vi "Encoder Init.vi"(0 "Portas":T1={"Acionador"="Dev1/port0/line7", "Clock"="Dev1/ctr0", "Canal Analogico"="Dev1/ai22", "Trigger"="/Dev1/PFI11"}) -> (3 "Task Out":T2, 6 "error out":errorcluster)   [LabVIEW 2019]
uses:
  <vilib>/DAQmx/create/channels.llb/DAQmx Create Channel (AI-Voltage-Basic).vi
  <vilib>/DAQmx/configure/timing.llb/DAQmx Timing (Sample Clock).vi
  <vilib>/DAQmx/create/channels.llb/DAQmx Create Channel (CO-Pulse Generation-Frequency).vi
  <vilib>/DAQmx/configure/timing.llb/DAQmx Timing (Implicit).vi
  <vilib>/DAQmx/create/channels.llb/DAQmx Create Channel (DO-Digital Output).vi
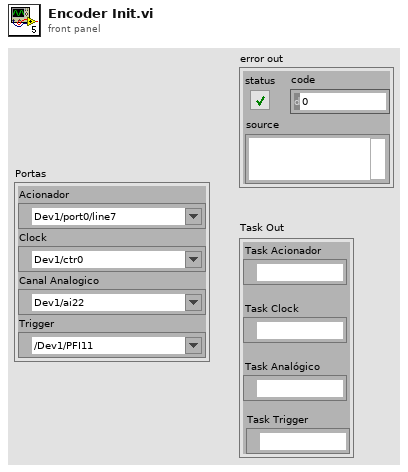
[diagram p1: front panel]
types:
  T1 = cluster{"Acionador":tag, "Clock":tag, "Canal Analogico":tag, "Trigger":tag}
  T2 = cluster{"Task Analógico":refnum<k21>, "Task Clock":refnum<k21>, "Task Acionador":refnum<k21>, "Task Trigger":tag}
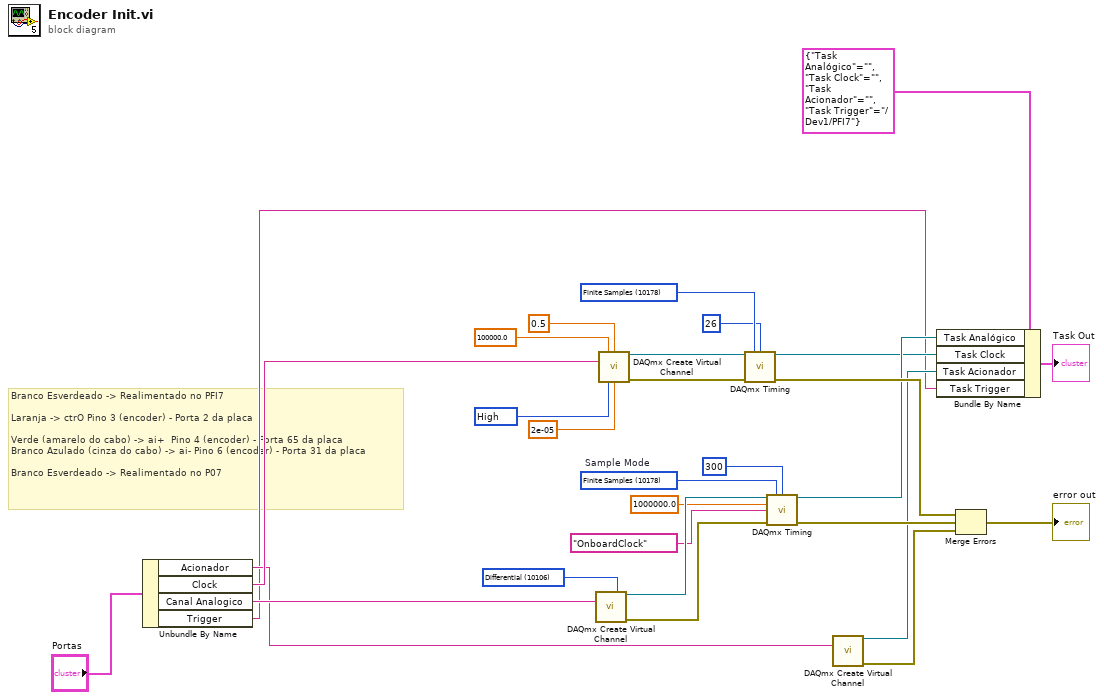
[diagram p0: block diagram]
diagram:
  w26 = 10106 items=["default"=-1, "RSE"=10083, "NRSE"=10078, "Differential"=10106, "Pseudodifferential"=12529] ("Terminal Configuration")
  w29 = 10178 items=["Finite Samples"=10178, "Continuous Samples"=10123, "Hardware Timed Single Point"=12522]  # Sample Mode
  w15 = 10192 items=["High"=10192, "Low"=10214] ("idle state")
  w20 = 10178 items=["Finite Samples"=10178, "Continuous Samples"=10123] ("sample mode")
  # "Branco Esverdeado -> Realimentado no PFI7\n\nLaranja -> ctrO Pino 3 (encoder) - Porta 2 da placa\n\nVerde (amarelo do cabo) -> ai+  Pino 4 (encoder) - Porta 65 da placa\nBranco Azulado (cinza do cabo) -> ai- Pino 6 (encoder) - Porta 31 da placa\n\nBranco Esverdeado -> Realimentado no P07"
  n1 = Unbundle By Name("Portas") -> ("Acionador"=w12:tag, "Clock"=w13:tag, "Canal Analogico"=w14:tag, "Trigger"=w1:tag)
  n2 = call-poly <vilib>:"DAQmx Create Virtual Channel.vi"("input terminal configuration"=w26, "physical channels"=w14) -> ("task out"=w27:refnum<k21>, "error out"=w28:errorcluster)  [unwired: 12 in]
  n3 = call-poly <vilib>:"DAQmx Create Virtual Channel.vi"("frequency"=100000.0, "duty cycle"=0.5, "counter"=w13, "idle state"=w15, "initial delay"=2e-05) -> ("task out"=w21:refnum<k21>, "error out"=w22:errorcluster)  [unwired: 9 in]
  n4 = call-poly <vilib>:"DAQmx Timing.vi"("task/channels in"=w21, "sample mode"=w20, "samples per channel"=26, "error in"=w22) -> ("task out"=w3:refnum<k21>, "error out"=w7:errorcluster)  [unwired: 10 in]
  n5 = call-poly <vilib>:"DAQmx Timing.vi"("task/channels in"=w27, "sample mode"=w29, "samples per channel"=300 ("Number of Samples"), "rate"=1000000.0 ("Sample Rate"), "source"=tag "OnboardClock" ("Sample Clock Source"), "error in"=w28) -> ("task out"=w4:refnum<k21>, "error out"=w8:errorcluster)  [unwired: 8 in]
  n6 = call-poly <vilib>:"DAQmx Create Virtual Channel.vi"("lines"=w12) -> ("task out"=w2:refnum<k21>, "error out"=w9:errorcluster)  [unwired: 13 in]
  n7 = Bundle By Name(cluster=T2 {"Task Analógico"="", "Task Clock"="", "Task Acionador"="", "Task Trigger"="/Dev1/PFI7"} ("Task Out 2"), "Task Analógico"=w4, "Task Clock"=w3, "Task Acionador"=w2, "Task Trigger"=w1) -> (→"Task Out":T2)
  n8 = Merge Errors(w7, w8, w9) -> (→"error out":errorcluster)
